vi "Configure User Defined Event (Condition).vi"(0 "VISA resource name":refnum<visa-resource-name>, 1 "Enable Inverse (F: Disable)":bool, 2 "Enable Condition Event (T: Enable)":bool=TRUE, 3 "Event Number (1)":i32=1 min=1 max=8 step=1, 5 "Condition (Empty)":string, 11 "error in (no error)":errorcluster) -> (4 "VISA resource name out":refnum<visa-resource-name>, 15 "error out":errorcluster)   [LabVIEW 2021, in "Yokogawa WT1800 Series.lvlib"]
doc: "Configures the user-defined events features, when the judgment condition specification method is Condition.\nSpecify judgment conditions using user-defined events."
uses:
  <instrlib>/Yokogawa WT1800 Series/Yokogawa WT1800 Series.lvlib
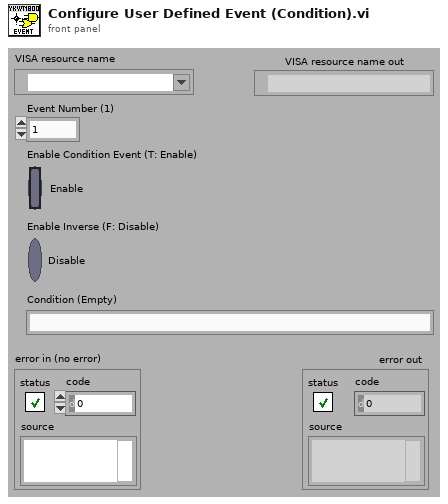
[diagram p1: front panel]
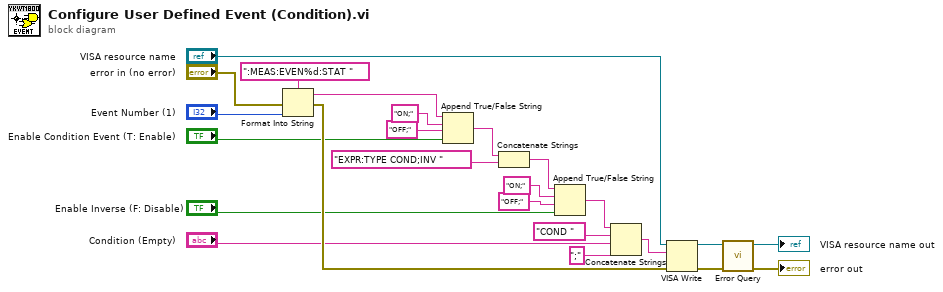
[diagram p0: block diagram]
diagram:
  n1 = Format Into String(format string=":MEAS:EVEN%d:STAT " ("形式文字列"), error in="error in (no error)", "Event Number (1)") -> (resulting string=w14:string, error out=w18:errorcluster)  [unwired: 1 in]
  n2 = Append True/False String ("True/False 文字列を追加")(1:"Enable Condition Event (T: Enable)", 2:"OFF;", 3:"ON;", 4:w14) -> (0:w11:string)
  n3 = Concatenate Strings(w11, "EXPR:TYPE COND;INV " ("文字列")) -> (w7:string)
  n4 = Append True/False String ("True/False 文字列を追加")(1:"Enable Inverse (F: Disable)", 2:"OFF;", 3:"ON;", 4:w7) -> (0:w4:string)
  n5 = Concatenate Strings(w4, "COND " ("文字列"), "Condition (Empty)", ";" ("文字列")) -> (w2:string)
  n6 = VISA Write ("VISA書き込み")(VISA resource name="VISA resource name", write buffer=w2, error in (no error)=w18) -> (VISA resource name out=w24:refnum<visa-resource-name>, error out=w23:errorcluster)  [unwired: 1 out]
  n7 = call <instrlib>:"Error Query.vi"("error in (no error)"=w23, "VISA resource name"=w24) -> ("error out"=→"error out":errorcluster, "VISA resource name out"=→"VISA resource name out":refnum<visa-resource-name>)  [unwired: 6 in, 2 out]
